vi "Display Tree Item.vi"(8 "error in (no error)":errorcluster, 10 "Tag":string, 11 "Application Data in":T1) -> (0 "error out":errorcluster, 3 "Application Data out":T1)   [LabVIEW 2020, in "DSF Configuration Utility.lvlib"]
uses:
  DSF Configuration Utility.lvlib
  Includes/DSF Core.lvlibp/Classes/Configuration Session/Configuration Session.lvclass
  Includes/DSF Core.lvlibp/Typedefs/DSF Direction.ctl
  Includes/DSF Core.lvlibp
  Includes/DSF Core.lvlibp/Typedefs/DSF Timing Info.ctl
  Includes/DSF Core.lvlibp/Typedefs/DSF Settings Info.ctl
  Includes/DSF Core.lvlibp/Typedefs/DSF Data Type.ctl
  Includes/DSF Core.lvlibp/Typedefs/DSF Engine Channel Configuration.ctl
  Includes/DSF Core.lvlibp/Typedefs/DSF Engine Transfer Configuration.ctl
  Includes/DSF Core.lvlibp/Typedefs/DSF Timeout Behavior.ctl
  Includes/DSF Core.lvlibp/Typedefs/DSF Engine Transfer Group Configuration.ctl
  Item Tree/ID to Tree Items/Tree Item Type.ctl
  Includes/DSF Core.lvlibp/Typedefs/Core Channel Configuration.ctl
  Includes/DSF Core.lvlibp/Classes/Configuration/Core/Channel/Channel Configuration.lvclass
  Includes/DSF Core.lvlibp/Typedefs/Core Transfer Configuration.ctl
  Includes/DSF Core.lvlibp/Classes/Configuration/Core/Transfer/Transfer Configuration.lvclass
  Includes/DSF Core.lvlibp/Typedefs/Core Group Configuration.ctl
  Includes/DSF Core.lvlibp/Classes/Configuration/Core/Group/Group Configuration.lvclass
  Application Data.ctl
  View Mode.ctl
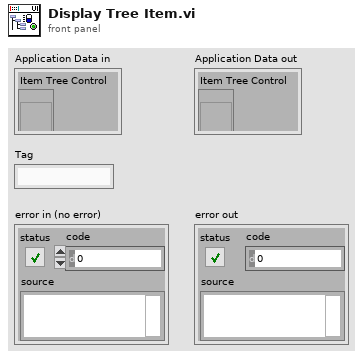
[diagram p1: front panel]
types:
  T1 = typedef "DSF Configuration Utility.lvlib/Application Data.ctl" = cluster{"Item Tree Control":refnum<vi>, "Value Tree Control":refnum<vi>, "Configuration Session":refnum<class "Configuration Session.lvclass">, "Top-Level VI":refnum<vi>, "View State":T2, "menu reference":refnum<k9>}
  T2 = typedef "DSF Configuration Utility.lvlib/View Mode.ctl" = enum16{"Tree", "List"}
  T3 = typedef "DSF Configuration Utility.lvlib/Tree Item Type.ctl" = enum16{"Plugin", "Group", "Transfer", "Channel", "Setting"}
  T4 = typedef "DSF Core.lvlibp/DSF Engine Transfer Group Configuration.ctl" = cluster{"core":T5, "component settings":T9[], "transfers":T10[]}
  T5 = typedef "DSF Core.lvlibp/Group Configuration.lvclass/Core Group Configuration.ctl" = cluster{"name":string, "direction":T6, "cycle timing":T7, "timeout behavior":T8, "enable conversion":bool}
  T6 = typedef "DSF Core.lvlibp/DSF Direction.ctl" = enum8{"Tx", "Rx"}
  T7 = typedef "DSF Core.lvlibp/DSF Timing Info.ctl" = cluster{"priority":u64, "decimation":u64, "offset":u64}
  T8 = typedef "DSF Core.lvlibp/DSF Timeout Behavior.ctl" = enum8{"Increment Late Count", "Throw Error"}
  T9 = typedef "DSF Core.lvlibp/DSF Settings Info.ctl" = cluster{"component":string, "values":cluster{"key":string, "value":string}[]}
  T10 = typedef "DSF Core.lvlibp/DSF Engine Transfer Configuration.ctl" = cluster{"core":T11, "component settings":T9[], "channels":T12[]}
  T11 = typedef "DSF Core.lvlibp/Transfer Configuration.lvclass/Core Transfer Configuration.ctl" = cluster{"name":string}
  T12 = typedef "DSF Core.lvlibp/DSF Engine Channel Configuration.ctl" = cluster{"core":T13, "component settings":T9[]}
  T13 = typedef "DSF Core.lvlibp/Channel Configuration.lvclass/Core Channel Configuration.ctl" = cluster{"name":string, "units":string, "engine data type":T14, "string data type":T14, "string offset":u64}
  T14 = typedef "DSF Core.lvlibp/DSF Data Type.ctl" = enum8{"Bool", "SGL", "DBL", "I8", "I16", "I32", "I64", "U8", "U16", "U32", "U64"}
  T15 = typedef "DSF Core.lvlibp/DSF Version Info.ctl" = cluster{"major":u32, "minor":u32, "fix":u32, "build":string}
  T16 = typedef "DSF Core.lvlibp/DSF Engine Plugin Configuration.ctl" = cluster{"name":string, "components":string[], "cycle timing":T7, "threads":T17[], "transfer groups":T19[], "settings":T18}
  T17 = typedef "DSF Core.lvlibp/DSF Engine Plugin Thread Configuration.ctl" = cluster{"processor":i32, "priority offset":i16, "settings":T18}
  T18 = typedef "DSF Core.lvlibp/DSF Settings Info.ctl" = cluster{"component":string, "name":string, "values":cluster{"key":string, "value":string}[]}[]
  T19 = typedef "DSF Core.lvlibp/DSF Engine Transfer Group Configuration.ctl" = cluster{"name":string, "direction":T6, "cycle timing":T7, "thread index":i32, "settings":T18, "transfers":T20[], "timeout behavior":T8}
  T20 = typedef "DSF Core.lvlibp/DSF Engine Transfer Configuration.ctl" = cluster{"name":string, "byte order":T21, "settings":T18, "channels":T22[]}
  T21 = typedef "DSF Core.lvlibp/DSF Byte Order.ctl" = enum8{"big-endian", "little-endian"}
  T22 = typedef "DSF Core.lvlibp/DSF Engine Channel Configuration.ctl" = cluster{"string offset":u64, "name":string, "units":string, "engine data type":T14, "string data type":T14, "settings":T18}
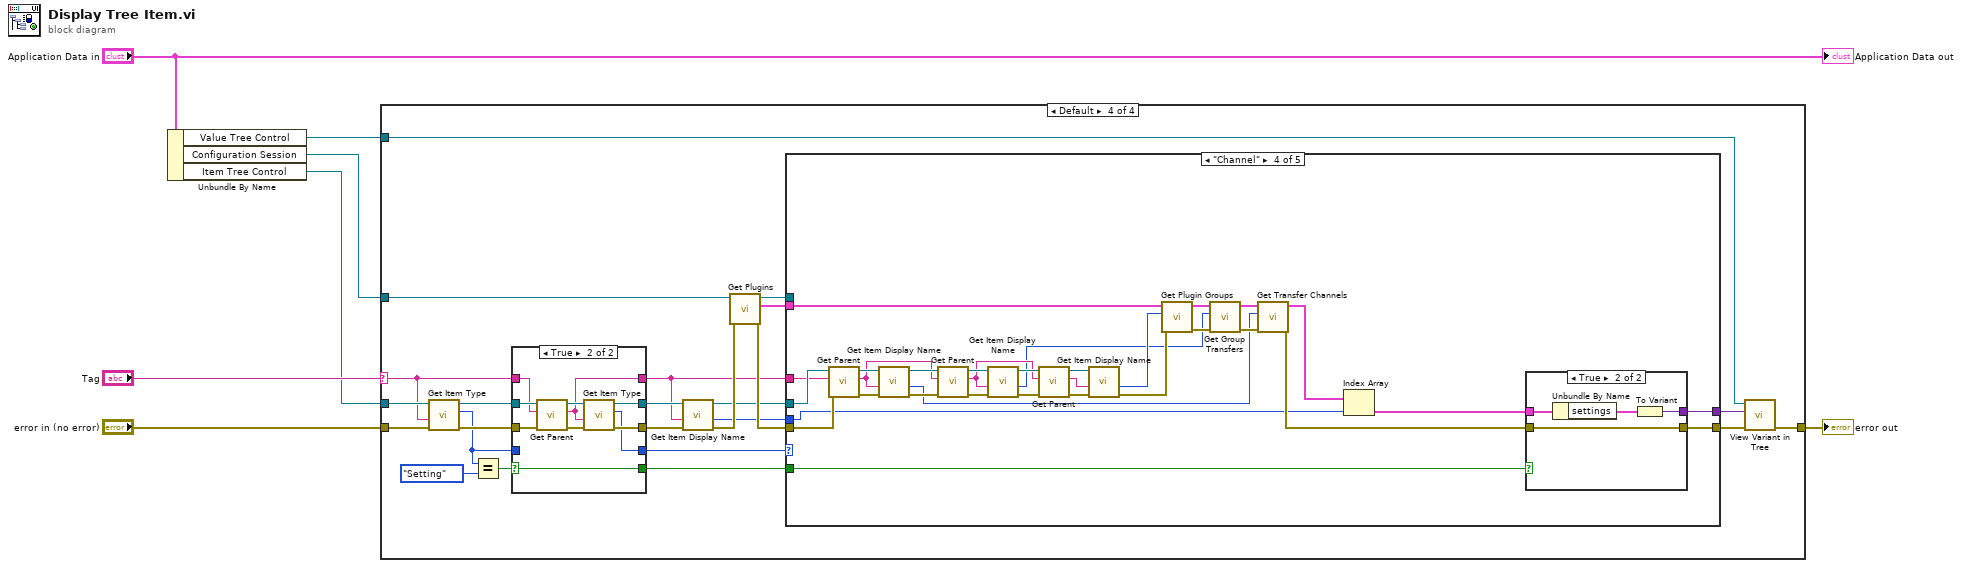
[diagram p0: block diagram]
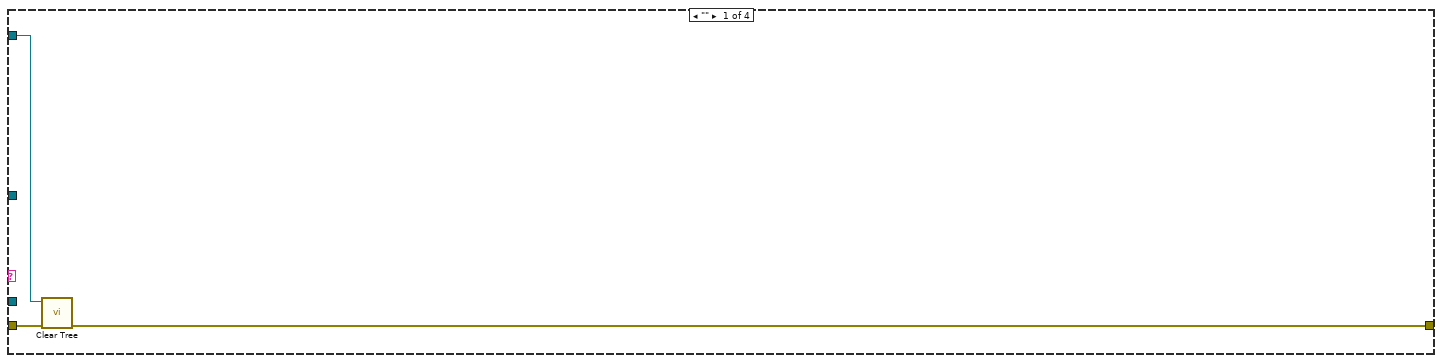
[diagram p2: hidden frame]
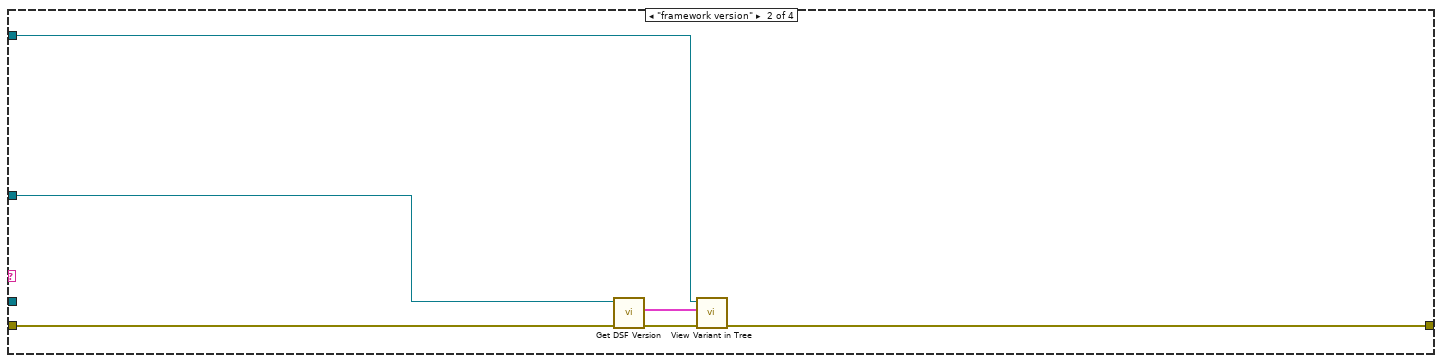
[diagram p3: hidden frame]
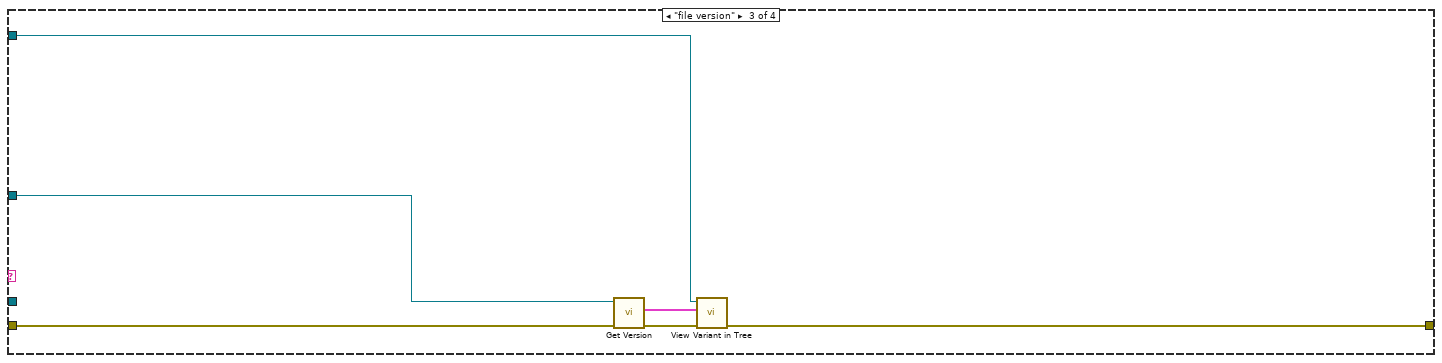
[diagram p4: hidden frame]
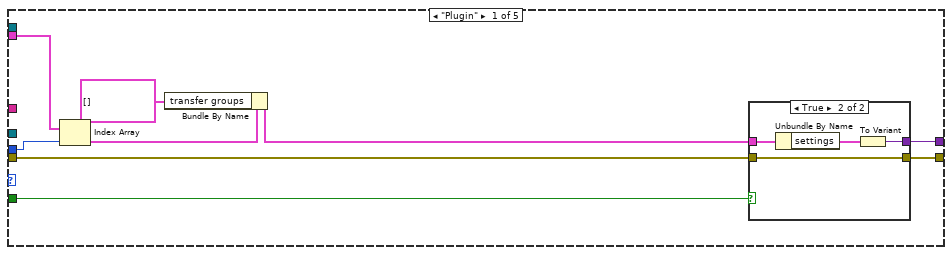
[diagram p6: hidden frame]
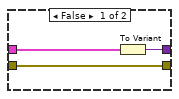
[diagram p7: hidden frame]
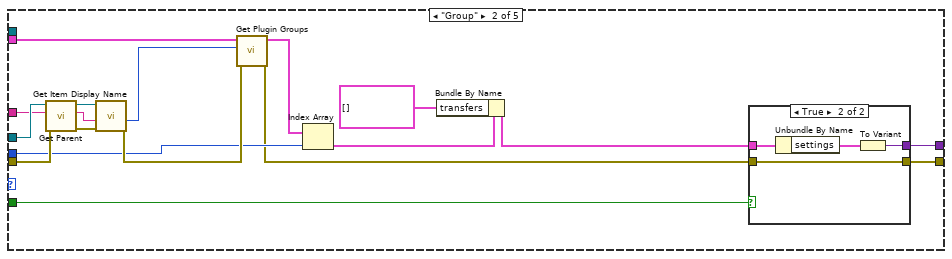
[diagram p8: hidden frame]
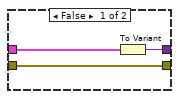
[diagram p9: hidden frame]
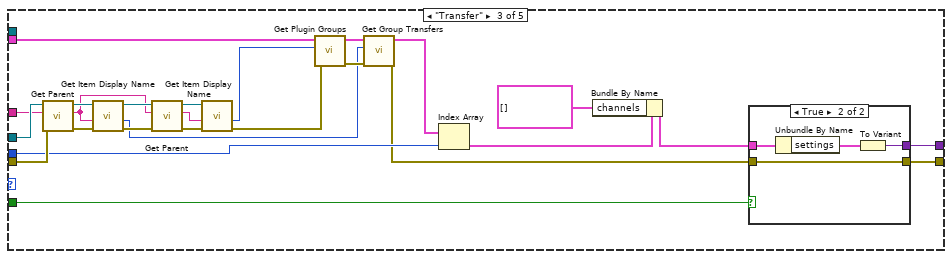
[diagram p10: hidden frame]
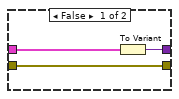
[diagram p11: hidden frame]
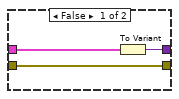
[diagram p12: hidden frame]
diagram:
  n1 = Unbundle By Name("Application Data in") -> ("Value Tree Control"=w1:refnum<vi>, "Configuration Session"=w6:refnum<class "Configuration Session.lvclass">, "Item Tree Control"=w5:refnum<vi>)
  n2 = case shown="Default" "Tag" {
    selector: "Tag" -> [_ _ _ w32]
    tunnel: w6 -> [_ w16 w22 w38]
    tunnel: w5 -> [_ _ _ w44]
    tunnel: "error in (no error)" -> [w10 w15 w21 w43]
    tunnel: w1 -> [w8 w12 w17 w35]
    tunnel: [w9 w13 w19 w41] -> w3
    frame "" {
      n3 = call "Clear Tree.vi"("error in (no error)"=w10, "TreeControl in"=w8) -> ("error out"=w9:errorcluster)  [unwired: 9 in]
    }
    frame "framework version" {
      n4 = call "Get DSF Version.vi"("error in (no error)"=w15, "configuration session in"=w16) -> ("error out"=w14:errorcluster, "dsf version"=w11:T15)  [unwired: 7 in, 1 out]
      n5 = call "View Variant in Tree.vi"("error in (no error)"=w14, "Variant"=w11, "TreeControl in"=w12) -> ("error out"=w13:errorcluster)  [unwired: 8 in]
    }
    frame "file version" {
      n6 = call "Get Version.vi"("error in (no error)"=w21, "configuration session in"=w22) -> ("error out"=w20:errorcluster, "version"=w18:T15)  [unwired: 7 in, 1 out]
      n7 = call "View Variant in Tree.vi"("error in (no error)"=w20, "Variant"=w18, "TreeControl in"=w17) -> ("error out"=w19:errorcluster)  [unwired: 8 in]
    }
    frame Default {
      n8 = call "Get Item Type.vi"("error in (no error)"=w43, "Tag"=w32, "TreeControl in"=w44) -> ("error out"=w30:errorcluster, "Item Type"=w27:T3, "TreeControl out"=w31:refnum<vi>)  [unwired: 6 in]
      n9 = Equal?(x=w27, y=Tree_Item_Type."Setting") -> (x = y?=w34:bool)
      n10 = case shown="True" w34 {
        selector: w34 -> [w47 w52]
        tunnel: w27 -> [w48 _]
        tunnel: w32 -> [w51 w54]
        tunnel: [w51 w53] -> w25
        tunnel: w31 -> [w49 w59]
        tunnel: w30 -> [w50 w58]
        tunnel: [w50 w57] -> w29
        tunnel: [w49 w56] -> w28
        tunnel: [w48 w55] -> w26
        tunnel: [w47 w52] -> w24
        frame False {
        }
        frame True {
          n11 = call "Get Parent.vi"("error in (no error)"=w58, "tag"=w54, "TreeControl in"=w59) -> ("error out"=w60:errorcluster, "parent tag"=w53:string, "TreeControl out"=w61:refnum<vi>)  [unwired: 5 in, 1 out]
          n12 = call "Get Item Type.vi"("error in (no error)"=w60, "Tag"=w53, "TreeControl in"=w61) -> ("error out"=w57:errorcluster, "Item Type"=w55:T3, "TreeControl out"=w56:refnum<vi>)  [unwired: 6 in]
        }
      }
      n13 = call "Get Item Display Name.vi"("error in (no error)"=w29, "Tag"=w25, "TreeControl in"=w28) -> ("error out"=w45:errorcluster, "index"=w39:i32, "TreeControl out"=w40:refnum<vi>)  [unwired: 5 in, 1 out]
      n14 = call "Get Plugins.vi"("error in (no error)"=w45, "configuration session in"=w38) -> ("error out"=w46:errorcluster, "plugins"=w36:T16[], "configuration session out"=w37:refnum<class "Configuration Session.lvclass">)  [unwired: 7 in]
      n15 = case shown="\"Channel\"" w26 {
        tunnel: [w65 w82 w107 w142 w175] -> w42
        tunnel: w46 -> [w64 w95 w128 w167 w175]
        tunnel: w37 -> [_ _ _ _ _]
        tunnel: [w62 w80 w106 w140 _] -> w23
        tunnel: w25 -> [_ w93 w126 w165 _]
        tunnel: w40 -> [_ w94 w127 w166 _]
        tunnel: w39 -> [w69 w86 w122 w137 _]
        tunnel: w36 -> [w70 w89 w123 w162 _]
        tunnel: w24 -> [w63 w78 w103 w139 _]
        frame "Plugin" {
          n16 = Index Array(array=w70, index=w69) -> (element=w68:T16)
          n17 = Bundle By Name(cluster=w68, "transfer groups"=T4[] []) -> (w66:T16)
          n18 = case shown="True" w63 {
            tunnel: w66 -> [w71 w76]
            tunnel: [w73 w77] -> w65
            tunnel: w64 -> [w73 w77]
            tunnel: [w72 w75] -> w62
            frame False {
              n19 = To Variant(anything=w71) -> (Variant=w72:variant)
            }
            frame True {
              n20 = Unbundle By Name(w76) -> ("settings"=w74:T18)
              n21 = To Variant(anything=w74) -> (Variant=w75:variant)
            }
          }
        }
        frame "Group" {
          n22 = call "Get Parent.vi"("error in (no error)"=w95, "tag"=w93, "TreeControl in"=w94) -> ("error out"=w91:errorcluster, "parent tag"=w90:string, "TreeControl out"=w92:refnum<vi>)  [unwired: 5 in, 1 out]
          n23 = call "Get Item Display Name.vi"("error in (no error)"=w91, "Tag"=w90, "TreeControl in"=w92) -> ("error out"=w88:errorcluster, "index"=w85:i32)  [unwired: 5 in, 2 out]
          n24 = call "Get Plugin Groups.vi"("error in (no error)"=w88, "plugin index"=w85, "plugins"=w89) -> ("error out"=w83:errorcluster, "transfer groups"=w87:T19[])  [unwired: 7 in]
          n25 = Index Array(array=w87, index=w86) -> (element=w79:T19)
          n26 = Bundle By Name(cluster=w79, "transfers"=T10[] []) -> (w81:T19)
          n27 = case shown="True" w78 {
            tunnel: w81 -> [w96 w101]
            tunnel: [w98 w102] -> w82
            tunnel: w83 -> [w98 w102]
            tunnel: [w97 w100] -> w80
            frame False {
              n28 = To Variant(anything=w96) -> (Variant=w97:variant)
            }
            frame True {
              n29 = Unbundle By Name(w101) -> ("settings"=w99:T18)
              n30 = To Variant(anything=w99) -> (Variant=w100:variant)
            }
          }
        }
        frame "Transfer" {
          n31 = call "Get Parent.vi"("error in (no error)"=w128, "tag"=w126, "TreeControl in"=w127) -> ("error out"=w124:errorcluster, "parent tag"=w116:string, "TreeControl out"=w125:refnum<vi>)  [unwired: 5 in, 1 out]
          n32 = call "Get Item Display Name.vi"("error in (no error)"=w124, "Tag"=w116, "TreeControl in"=w125) -> ("error out"=w115:errorcluster, "index"=w110:i32, "TreeControl out"=w117:refnum<vi>)  [unwired: 5 in, 1 out]
          n33 = call "Get Parent.vi"("error in (no error)"=w115, "tag"=w116, "TreeControl in"=w117) -> ("error out"=w114:errorcluster, "parent tag"=w111:string, "TreeControl out"=w118:refnum<vi>)  [unwired: 5 in, 1 out]
          n34 = call "Get Item Display Name.vi"("error in (no error)"=w114, "Tag"=w111, "TreeControl in"=w118) -> ("error out"=w113:errorcluster, "index"=w112:i32)  [unwired: 5 in, 2 out]
          n35 = call "Get Plugin Groups.vi"("error in (no error)"=w113, "plugin index"=w112, "plugins"=w123) -> ("error out"=w119:errorcluster, "transfer groups"=w121:T19[])  [unwired: 7 in]
          n36 = call "Get Group Transfers.vi"("error in (no error)"=w119, "group index"=w110, "transfer groups"=w121) -> ("error out"=w105:errorcluster, "transfers"=w120:T20[])  [unwired: 7 in]
          n37 = Index Array(array=w120, index=w122) -> (element=w108:T20)
          n38 = Bundle By Name(cluster=w108, "channels"=T12[] []) -> (w104:T20)
          n39 = case shown="True" w103 {
            tunnel: w104 -> [w129 w134]
            tunnel: [w131 w135] -> w107
            tunnel: w105 -> [w131 w135]
            tunnel: [w130 w133] -> w106
            frame False {
              n40 = To Variant(anything=w129) -> (Variant=w130:variant)
            }
            frame True {
              n41 = Unbundle By Name(w134) -> ("settings"=w132:T18)
              n42 = To Variant(anything=w132) -> (Variant=w133:variant)
            }
          }
        }
        frame "Channel" {
          n43 = call "Get Parent.vi"("error in (no error)"=w167, "tag"=w165, "TreeControl in"=w166) -> ("error out"=w163:errorcluster, "parent tag"=w157:string, "TreeControl out"=w164:refnum<vi>)  [unwired: 5 in, 1 out]
          n44 = call "Get Item Display Name.vi"("error in (no error)"=w163, "Tag"=w157, "TreeControl in"=w164) -> ("error out"=w156:errorcluster, "index"=w146:i32, "TreeControl out"=w158:refnum<vi>)  [unwired: 5 in, 1 out]
          n45 = call "Get Parent.vi"("error in (no error)"=w156, "tag"=w157, "TreeControl in"=w158) -> ("error out"=w155:errorcluster, "parent tag"=w144:string, "TreeControl out"=w159:refnum<vi>)  [unwired: 5 in, 1 out]
          n46 = call "Get Item Display Name.vi"("error in (no error)"=w155, "Tag"=w144, "TreeControl in"=w159) -> ("error out"=w147:errorcluster, "index"=w136:i32, "TreeControl out"=w148:refnum<vi>)  [unwired: 5 in, 1 out]
          n47 = call "Get Parent.vi"("error in (no error)"=w147, "tag"=w144, "TreeControl in"=w148) -> ("error out"=w150:errorcluster, "parent tag"=w151:string, "TreeControl out"=w149:refnum<vi>)  [unwired: 5 in, 1 out]
          n48 = call "Get Item Display Name.vi"("error in (no error)"=w150, "Tag"=w151, "TreeControl in"=w149) -> ("error out"=w145:errorcluster, "index"=w138:i32)  [unwired: 5 in, 2 out]
          n49 = call "Get Plugin Groups.vi"("error in (no error)"=w145, "plugin index"=w138, "plugins"=w162) -> ("error out"=w160:errorcluster, "transfer groups"=w161:T19[])  [unwired: 7 in]
          n50 = call "Get Group Transfers.vi"("error in (no error)"=w160, "group index"=w136, "transfer groups"=w161) -> ("error out"=w153:errorcluster, "transfers"=w154:T20[])  [unwired: 7 in]
          n51 = call "Get Transfer Channels.vi"("error in (no error)"=w153, "transfer index"=w146, "transfers"=w154) -> ("error out"=w143:errorcluster, "channels"=w152:T22[])  [unwired: 7 in]
          n52 = Index Array(array=w152, index=w137) -> (element=w141:T22)
          n53 = case shown="True" w139 {
            tunnel: w141 -> [w168 w173]
            tunnel: [w170 w174] -> w142
            tunnel: w143 -> [w170 w174]
            tunnel: [w169 w172] -> w140
            frame False {
              n54 = To Variant(anything=w168) -> (Variant=w169:variant)
            }
            frame True {
              n55 = Unbundle By Name(w173) -> ("settings"=w171:T18)
              n56 = To Variant(anything=w171) -> (Variant=w172:variant)
            }
          }
        }
        frame "Setting" {
        }
      }
      n57 = call "View Variant in Tree.vi"("error in (no error)"=w42, "Variant"=w23, "TreeControl in"=w35) -> ("error out"=w41:errorcluster)  [unwired: 8 in]
    }
  }
  "error out" <- w3
  "Application Data out" <- "Application Data in"
